vi "Load CD settings.vi"() -> ()   [LabVIEW 2019]
uses:
  Shared/Compiled.Settings.ctl
  Shared/main_page_config.ctl
  Shared/object_managament_config.ctl
  Shared/interaction_parameter_configuration.ctl
  Shared/object_attribute_configuration.ctl
  Shared/object_status_info.ctl
  Shared/object_data.ctl
  <vilib>/NI VeriStand/Custom Device API/Block Data Reference.ctl
  <vilib>/NI VeriStand/Custom Device API/Data Reference.ctl
  Shared/HLA Custom Device Shared.lvlib
  <vilib>/NI VeriStand/Custom Device API/Custom Device API.lvlib
panel:
  out "data":T1={"Name"="HLA Custom Device", "Async Init Timeout"=10000, "target main properties"={"Federate Execution Name"="MAKsimple", "Federate Type"="niveristand", "Local Designator Settings"="", "FOM Module"=path "/usr/local/mak/makRti4.6/bin/MAKsimple1516e.xml", "mak mtl file"=path "c:/ni-rt/NIVeriStand/testDev_force_manual.mtl", "FOM destination path"="/usr/local/mak/makRti4.6/bin", "MTL destination path"=""}, "obiectConfig"={"incoming interactions"=[{"interaction class name"="WeaponFire", "parameter name"="FuseType", "datatype"="c", "vsChIndex"=3, "vsObjectId"=""}, {"interaction class name"="WeaponFire", "parameter name"="RateOfFire", "datatype"="e", "vsChIndex"=4, "vsObjectId"=""}], "incoming objects"=[], "outgoing interactions"=[], "outgoing objects"=[]}, "objectStatus"={"incoming interactions"={"WeaponFire"={"OrderType"=1, "Timestamp"=0, "TransportType"=2}}, "incoming objects"={"BaseEntity_0"={"Attributes"=4, "InstanceID"=3, "OrderType"=1, "Timestamp"=0, "TransportType"=2}}, "outgoing interactions"={}, "outgoing objects"={}}, "objectData"={"out interaction data BD"=[], "out interaction data size"=0, "out interaction status BD"=[], "out interaction status size"=0, "out object data BD"=[], "out object data size"=0, "out object status BD"=[], "out object status size"=0}} {"objectData"."out object status BD"."Data Reference" format="%.0x"; "objectData"."out object data BD"."Data Reference" format="%.0x"; "objectData"."out interaction status BD"."Data Reference" format="%.0x"; "objectData"."out interaction data BD"."Data Reference" format="%.0x"}
  in  "file (use dialog)":path=path "C:/Users/Administrator/Documents/LabVIEW Data/cdsettings.bin"
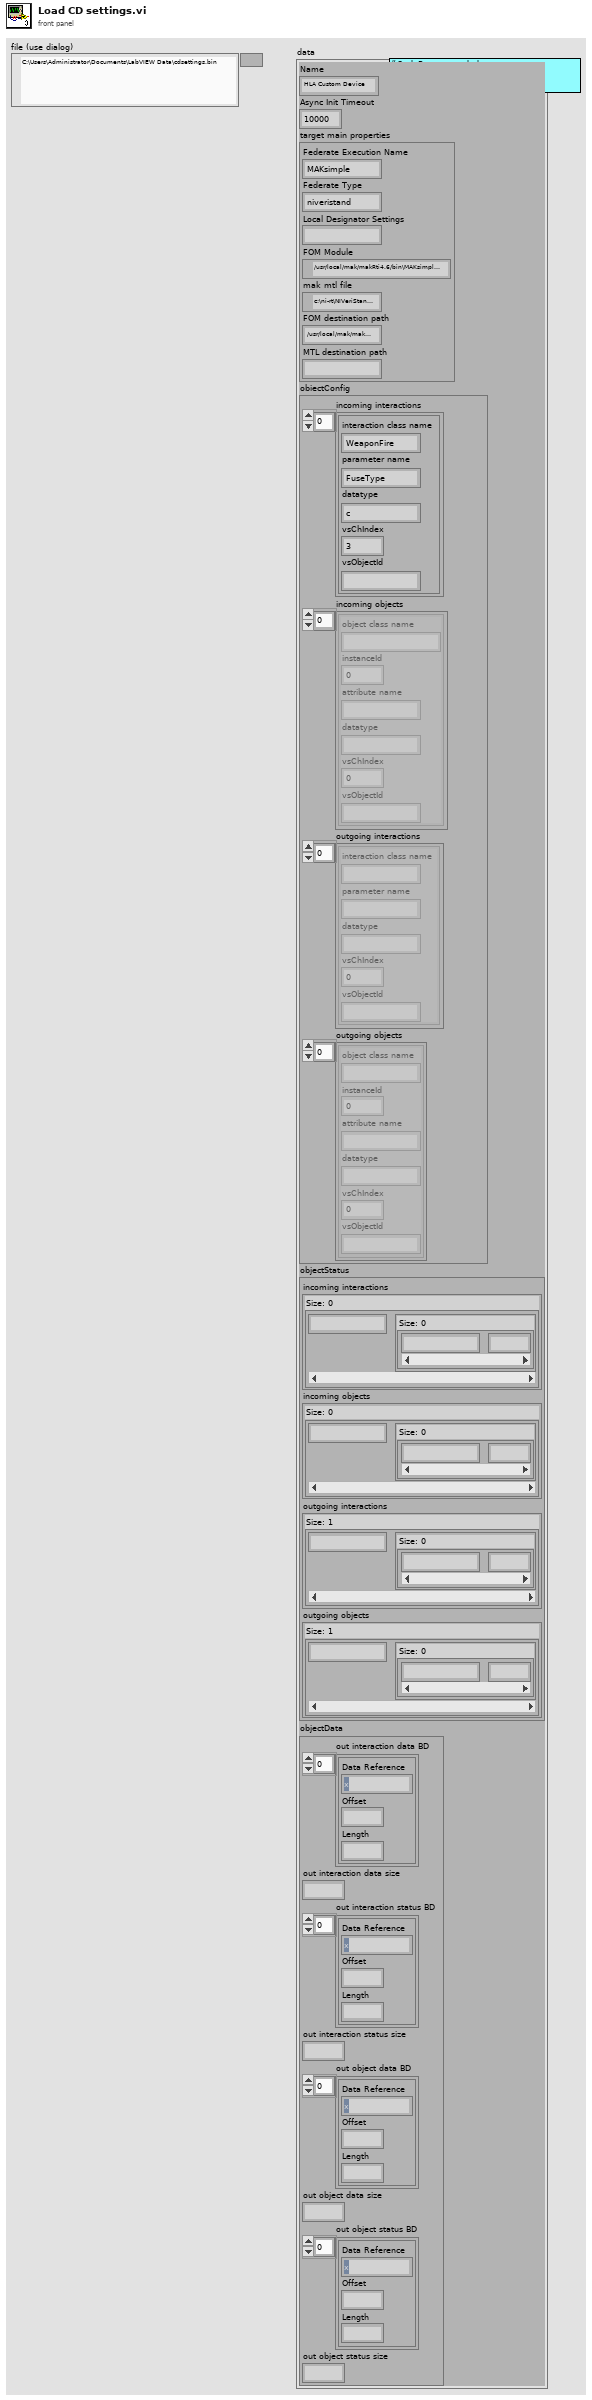
[diagram p1: front panel]
types:
  T1 = typedef "HLA Custom Device Shared.lvlib/Compiled.Settings.ctl" = cluster{"Name":string, "Async Init Timeout":u16, "target main properties":T2, "obiectConfig":T3, "objectStatus":T6, "objectData":T7}
  T2 = typedef "HLA Custom Device Shared.lvlib/main_page_config.ctl" = cluster{"Federate Execution Name":string, "Federate Type":string, "Local Designator Settings":string, "FOM Module":path, "mak mtl file":path, "FOM destination path":string, "MTL destination path":string}
  T3 = typedef "HLA Custom Device Shared.lvlib/object_managament_config.ctl" = cluster{"incoming interactions":T4[], "incoming objects":T5[], "outgoing interactions":T4[], "outgoing objects":T5[]}
  T4 = typedef "HLA Custom Device Shared.lvlib/interaction_parameter_configuration.ctl" = cluster{"interaction class name":string, "parameter name":string, "datatype":string, "vsChIndex":i32, "vsObjectId":string}
  T5 = typedef "HLA Custom Device Shared.lvlib/object_attribute_configuration.ctl" = cluster{"object class name":string, "instanceId":i32, "attribute name":string, "datatype":string, "vsChIndex":i32, "vsObjectId":string}
  T6 = typedef "HLA Custom Device Shared.lvlib/object_status_info.ctl" = cluster{"incoming interactions":map{string, map{string, i32}}, "incoming objects":map{string, map{string, i32}}, "outgoing interactions":map{string, map{string, i32}}, "outgoing objects":map{string, map{string, i32}}}
  T7 = typedef "HLA Custom Device Shared.lvlib/object_data.ctl" = cluster{"out interaction data BD":T8[], "out interaction data size":i32, "out interaction status BD":T8[], "out interaction status size":i32, "out object data BD":T8[], "out object data size":i32, "out object status BD":T8[], "out object status size":i32}
  T8 = typedef "Custom Device API.lvlib/Block Data Reference.ctl" = cluster{"Data Reference":T9, "Offset":u64, "Length":u64}
  T9 = typedef "Custom Device API.lvlib/Data Reference.ctl" = i32
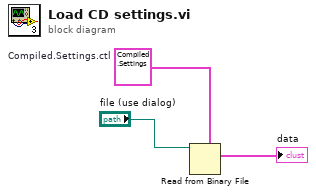
[diagram p0: block diagram]
diagram:
  w2 = T1 {"Name"="", "Async Init Timeout"=0, "target main properties"={"Federate Execution Name"="", "Federate Type"="", "Local Designator Settings"="", "FOM Module"=path "", "mak mtl file"=path "", "FOM destination path"="", "MTL destination path"=""}, "obiectConfig"={"incoming interactions"=[], "incoming objects"=[], "outgoing interactions"=[], "outgoing objects"=[]}, "objectStatus"={"incoming interactions"={}, "incoming objects"={}, "outgoing interactions"={}, "outgoing objects"={}}, "objectData"={"out interaction data BD"=[], "out interaction data size"=0, "out interaction status BD"=[], "out interaction status size"=0, "out object data BD"=[], "out object data size"=0, "out object status BD"=[], "out object status size"=0}}  # Compiled.Settings.ctl
  n1 = Read from Binary File(5:w2, 11:"file (use dialog)") -> (2:→"data":T1)  [unwired: 4 in, 3 out]
